vi "TimeStampedToElapsedTimeMessage.vi"(10 "Time Opened":timestamp, 11 "TimeStampedMessage":T2) -> (3 "ElapsedTimeMessage":T1)   [LabVIEW 2012, in "NetworkStreamWriter.lvclass"]
doc: "Converts a messge with a time stamp to a message with an elapsed time since the last reconnection between the writer and its corresponding reader endpoint.\n\nJared Kirschner, 2012."
uses:
  NetworkStreamWriter.lvclass
  Shared/TimeStampedMessage.ctl
  Shared/ElapsedTimeMessage.ctl
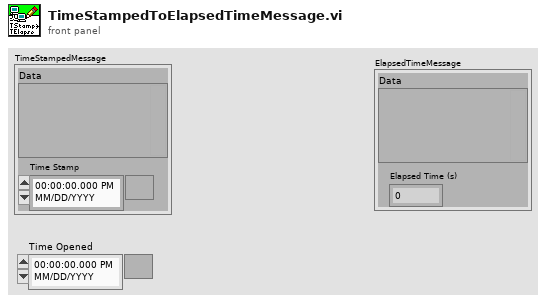
[diagram p1: front panel]
types:
  T1 = typedef "ElapsedTimeMessage.ctl" = cluster{"Data":variant, "Elapsed Time (s)":dbl}
  T2 = typedef "TimeStampedMessage.ctl" = cluster{"Data":variant, "Time Stamp":timestamp}
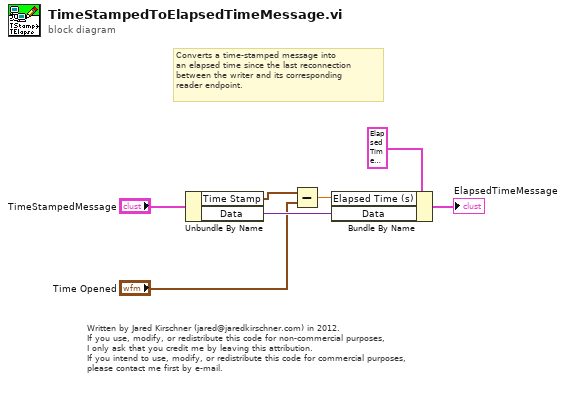
[diagram p0: block diagram]
diagram:
  # "Converts a time-stamped message into\nan elapsed time since the last reconnection\nbetween the writer and its corresponding \nreader endpoint."
  # "Written by Jared Kirschner (jared@jaredkirschner.com) in 2012.\nIf you use, modify, or redistribute this code for non-commercial purposes,\nI only ask that you credit me by leaving this attribution.\nIf you intend to use, modify, or redistribute this code for commercial purposes,\nplease contact me first by e-mail."
  n1 = Unbundle By Name("TimeStampedMessage") -> ("Time Stamp"=w5:timestamp, "Data"=w6:variant)
  n2 = Subtract(x=w5, y="Time Opened") -> (x-y=w4:dbl)
  n3 = Bundle By Name(cluster=T1 {"Data"=variant, "Elapsed Time (s)"=0.0} ("Message"), "Elapsed Time (s)"=w4, "Data"=w6) -> (→"ElapsedTimeMessage":T1)
